vi "createPW.vi"() -> (0 "String":string)   [LabVIEW 2012, in "HGF_GPG.lvlib" / "HGF_GPG.lvclass"]
doc: "creates a random password string\n\nF.Berck@gsi.de"
uses:
  HGF_GPG.lvclass
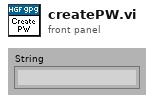
[diagram p1: front panel]
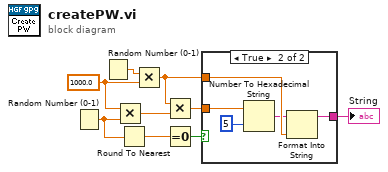
[diagram p0: block diagram]
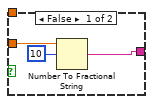
[diagram p2: hidden frame]
diagram:
  w6 = 1000.0 ("x")
  n1 = Random Number (0-1)() -> (number: 0 to 1=w4:dbl)
  n2 = Random Number (0-1)() -> (number: 0 to 1=w3:dbl)
  n3 = Multiply(x=w6, y=w4) -> (x*y=w5:dbl)
  n4 = Round To Nearest(number=w4) -> (nearest integer value=w1:dbl)
  n5 = Multiply(x=w3, y=w6) -> (x*y=w8:dbl)
  n6 = Multiply(x=w8, y=w5) -> (x*y=w7:dbl)
  n7 = Equal To 0?(x=w1) -> (x = 0?=w2:bool)
  n8 = case shown="True" w2 {
    tunnel: [w11 w13] -> w9
    tunnel: w7 -> [w10 w16]
    tunnel: w8 -> [_ w15]
    frame False {
      n9 = Number To Fractional String(number=w10, width (-)=i16 10) -> (F-format string=w11:string)  [unwired: 2 out]
    }
    frame True {
      n10 = Number To Hexadecimal String(1:i16 5 ("width (-)"), 2:w16) -> (0:w14:string)
      n11 = Format Into String(initial string=w14, w15) -> (resulting string=w13:string)  [unwired: 2 in, 1 out]
    }
  }
  "String" <- w9
